vi "执行.vi"(8 "error in (no error)":errorcluster caption="错误输入（无错误）", 11 "命令：关闭照明灯 输入":refnum<class "命令：关闭照明灯.lvclass"> caption="DNL_LabVIEW Object in") -> (0 "error out":errorcluster caption="错误输出", 3 "命令：关闭照明灯 输出":refnum<class "命令：关闭照明灯.lvclass"> caption="DNL_LabVIEW Object out")   [LabVIEW 2011, in "命令：关闭照明灯.lvclass"]
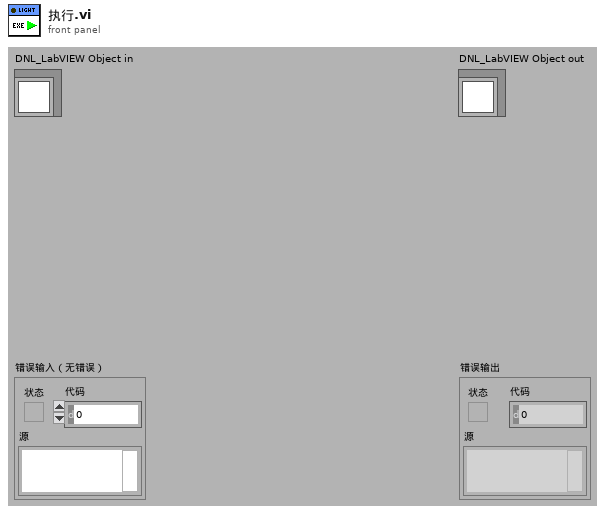
[diagram p1: front panel]
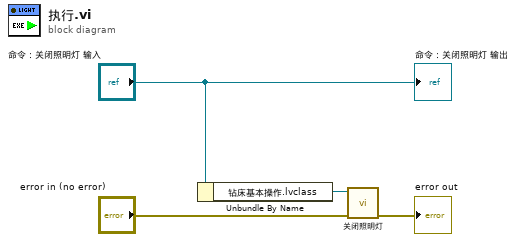
[diagram p0: block diagram]
diagram:
  n1 = Unbundle By Name("命令：关闭照明灯 输入") -> ("钻床基本操作.lvclass"=w3:refnum<class "钻床基本操作.lvclass">)
  n2 = call "关闭照明灯.vi"("error in (no error)"="error in (no error)", "钻床基本操作 输入"=w3) -> ("error out"=→"error out":errorcluster)  [unwired: 8 in, 1 out]
  "命令：关闭照明灯 输出" <- "命令：关闭照明灯 输入"
